vi "Write Inputs.vi"(8 "error in (no error)":errorcluster, 10 "Inputs":T1[](array[typedef]), 11 "CallVIStep in":refnum<class "CallVIStep.lvclass">) -> (0 "error out":errorcluster, 3 "CallVIStep out":refnum<class "CallVIStep.lvclass">)   [LabVIEW 2015, in "CallVIStep.lvclass"]
uses:
  CallVIStep.lvclass
  VI Input Typedef.ctl
  VI Input Type Typedef.ctl
  CallVIStep.lvclass/CallVIStep.ctl
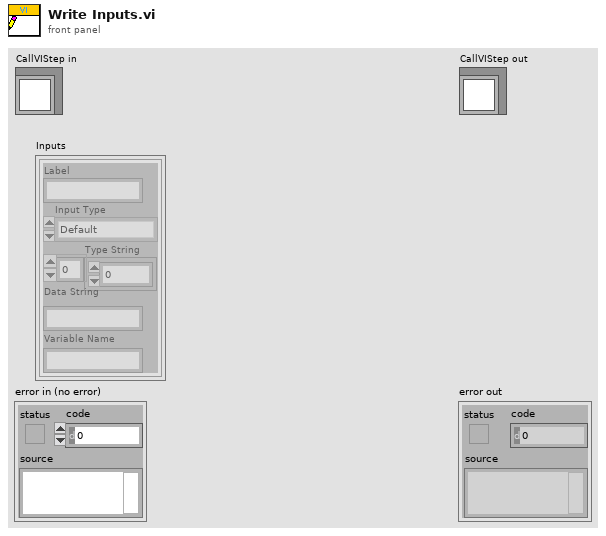
[diagram p1: front panel]
types:
  T1 = typedef "CallVIStep.lvclass/VI Input Typedef.ctl" = cluster{"Label":string, "Input Type":T2, "Type String":i16[], "Data String":string, "Variable Name":string}
  T2 = typedef "CallVIStep.lvclass/VI Input Type Typedef.ctl" = enum16{"Default", "Value", "Variable"}
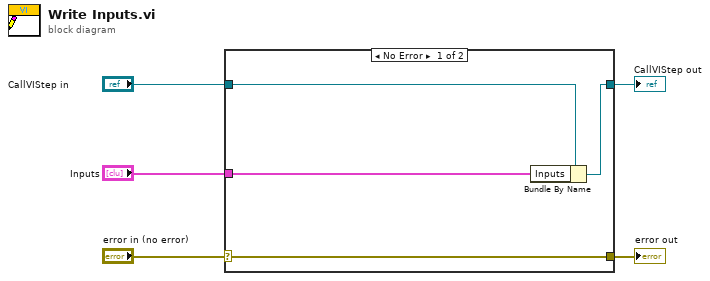
[diagram p0: block diagram]
diagram:
  n1 = case shown="No Error" "error in (no error)" {
    selector: "error in (no error)" -> [w9 w10]
    tunnel: [w9 w10] -> w4
    tunnel: [w7 w11] -> w2
    tunnel: "CallVIStep in" -> [w8 w11]
    tunnel: "Inputs" -> [w6 _]
    frame No Error {
      n2 = Bundle By Name(cluster=w8, "Inputs"=w6) -> (w7:refnum<class "CallVIStep.lvclass">)
    }
    frame Error {
    }
  }
  "error out" <- w4
  "CallVIStep out" <- w2
